vi "PhidgetDisableServerDiscovery.vi"(8 "error in":errorcluster) -> (0 "error out":errorcluster)   [LabVIEW 2012, in "Phidget Common.lvlib"]
doc: "${DisableServerDiscovery:Header}"
uses:
  <instrlib>/Phidgets/Phidget Common/Phidget Common.lvlib
  phidget22.dll
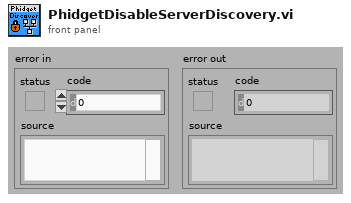
[diagram p1: front panel]
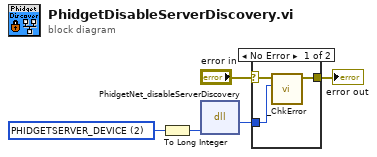
[diagram p0: block diagram]
diagram:
  w2 = u32 2 items=["PHIDGETSERVER_NONE", "PHIDGETSERVER_DEVICELISTENER", "PHIDGETSERVER_DEVICE", "PHIDGETSERVER_DEVICEREMOTE", "PHIDGETSERVER_DICTIONARYLISTENER", "PHIDGETSERVER_DICTIONARY", "PHIDGETSERVER_DICTIONARYREMOTE", "PHIDGETSERVER_WWWLISTENER", "PHIDGETSERVER_WWW", "PHIDGETSERVER_WWWREMOTE", "PHIDGETSERVER_SBC"] ("srvt")
  n1 = To Long Integer(number=w2) -> (32bit integer=w1:i32)
  n2 = dll-call lib="phidget22.dll" fn="PhidgetNet_disableServerDiscovery"("srvt"=w1) -> ("return type"=w3:i32)  [unwired: 4 in, 2 out]
  n3 = case shown="No Error" "error in" {
    selector: "error in" -> [w6 w9]
    tunnel: [w8 w9] -> w4
    tunnel: w3 -> [w7 _]
    frame No Error {
      n4 = call <instrlib>:"_ChkError.vi"("Return Code"=w7, "error in (no error)"=w6) -> ("error out"=w8:errorcluster)  [unwired: 9 in]
    }
    frame Error {
    }
  }
  "error out" <- w4
